vi "gyro -- sourcer async - V3 -- mfli.vi"(11 "sourcer event pair":T1) -> ()   [LabVIEW 2021]
uses:
  server talk-to-back pair.ctl
  server talkback message type.ctl
  server talkto message type.ctl
  mfli reader event.ctl
  MFLI frontend action.ctl
  publisher action.ctl
  data source action.ctl
  PLL data source.ctl
panel:
  in  "all":enum32{"all", "all 2"}(tab)
  out "read Voltage (V)":cdb=1e-323+8e-323i format="%#_6p"
  in  "read OK":bool
  out "read Voltage X (V)":dbl=1e-323 format="%#_6p"
  out "read Voltage Y (V)":dbl=8e-323 format="%#_6p"
  in  "delay-read (msec)":i64=20
  out "zi freq (Hz)":dbl=6.9251494997198e-310 format="%-#.3f"
  in  "amplitude (V)":dbl=0.001 format="%#_6p"
  in  "start  !":bool
  in  "stop  !":bool
  out "device selector":enum32{"MFLI"}(tab)
  in  "MFLI Address":string="DEV4307"
  in  "set amp!":bool
  in  "data rate (Sa/s)":dbl=100000.0 format="%#_6p"
  in  "set data rate!":bool
  in  "init MFLI addr !":bool
  out "Stopped?":bool=TRUE
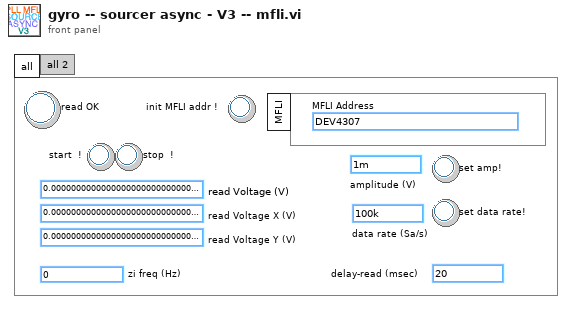
[diagram p1: front panel]
types:
  T1 = typedef "server talk-to-back pair.ctl" = cluster{"talkback event":refnum<user-event>, "talkto event":refnum<user-event>}
  T2 = typedef "MFLI frontend action.ctl" = enum16{"read", "writeread", "open", "close", "write"}
  T3 = typedef "server talkto message type.ctl" = cluster{"message":enum16{"stop", "start", "update pars", "update request", "new", "launch", "exit", "get", "reset", "pause", "unpause"}}
  T4 = typedef "mfli reader event.ctl" = enum16{"start", "stop", "exit", "set amplitude", "set datarate", "init"}
  T5 = typedef "Zurich Instruments LabOne.lvlib/ziTypeHandle.ctl" = cluster{"handleValid":bool, "Conn":u64, "Path Prefix":string, "Handle":u64, "Connected":bool, "Clockbase(s)":dbl}
  T6 = typedef "publisher action.ctl" = enum16{"set", "get", "init", "check"}
  T7 = typedef "PLL data source.ctl" = enum16{"meta", "MFLI", "SRS865A", "arydh"}
  T8 = typedef "data source action.ctl" = enum16{"set", "get", "init", "set-and-get", "init source"}
  T9 = typedef "eventvkey.ctl" = enum16{"ASCII", "Enter", "Return", "Shift", "Ctrl", "Alt", "Cmd", "Opt", "Caps", "NumLock", "Clear", "Break", "Up", "Down", "Left", "Right", "Insert", "Delete", "Home", "End", "PageUp", "PageDown", "Escape", "Help", "Pause", "ScrollLock", "F1", "F2", "F3", "F4", "F5", "F6", "F7", "F8", "F9", "F10", "F11", "F12", "F13", "F14", "F15", "F16", "F17", "F18", "F19", "F20", "F21", "F22", "F23", "F24", "Play", "VolumeUp", "VolumeDown", "Mute", "Two Byte Char"}
  T10 = enum16{"stop", "start", "update pars", "update request", "new", "launch", "exit", "get", "reset", "pause", "unpause"}
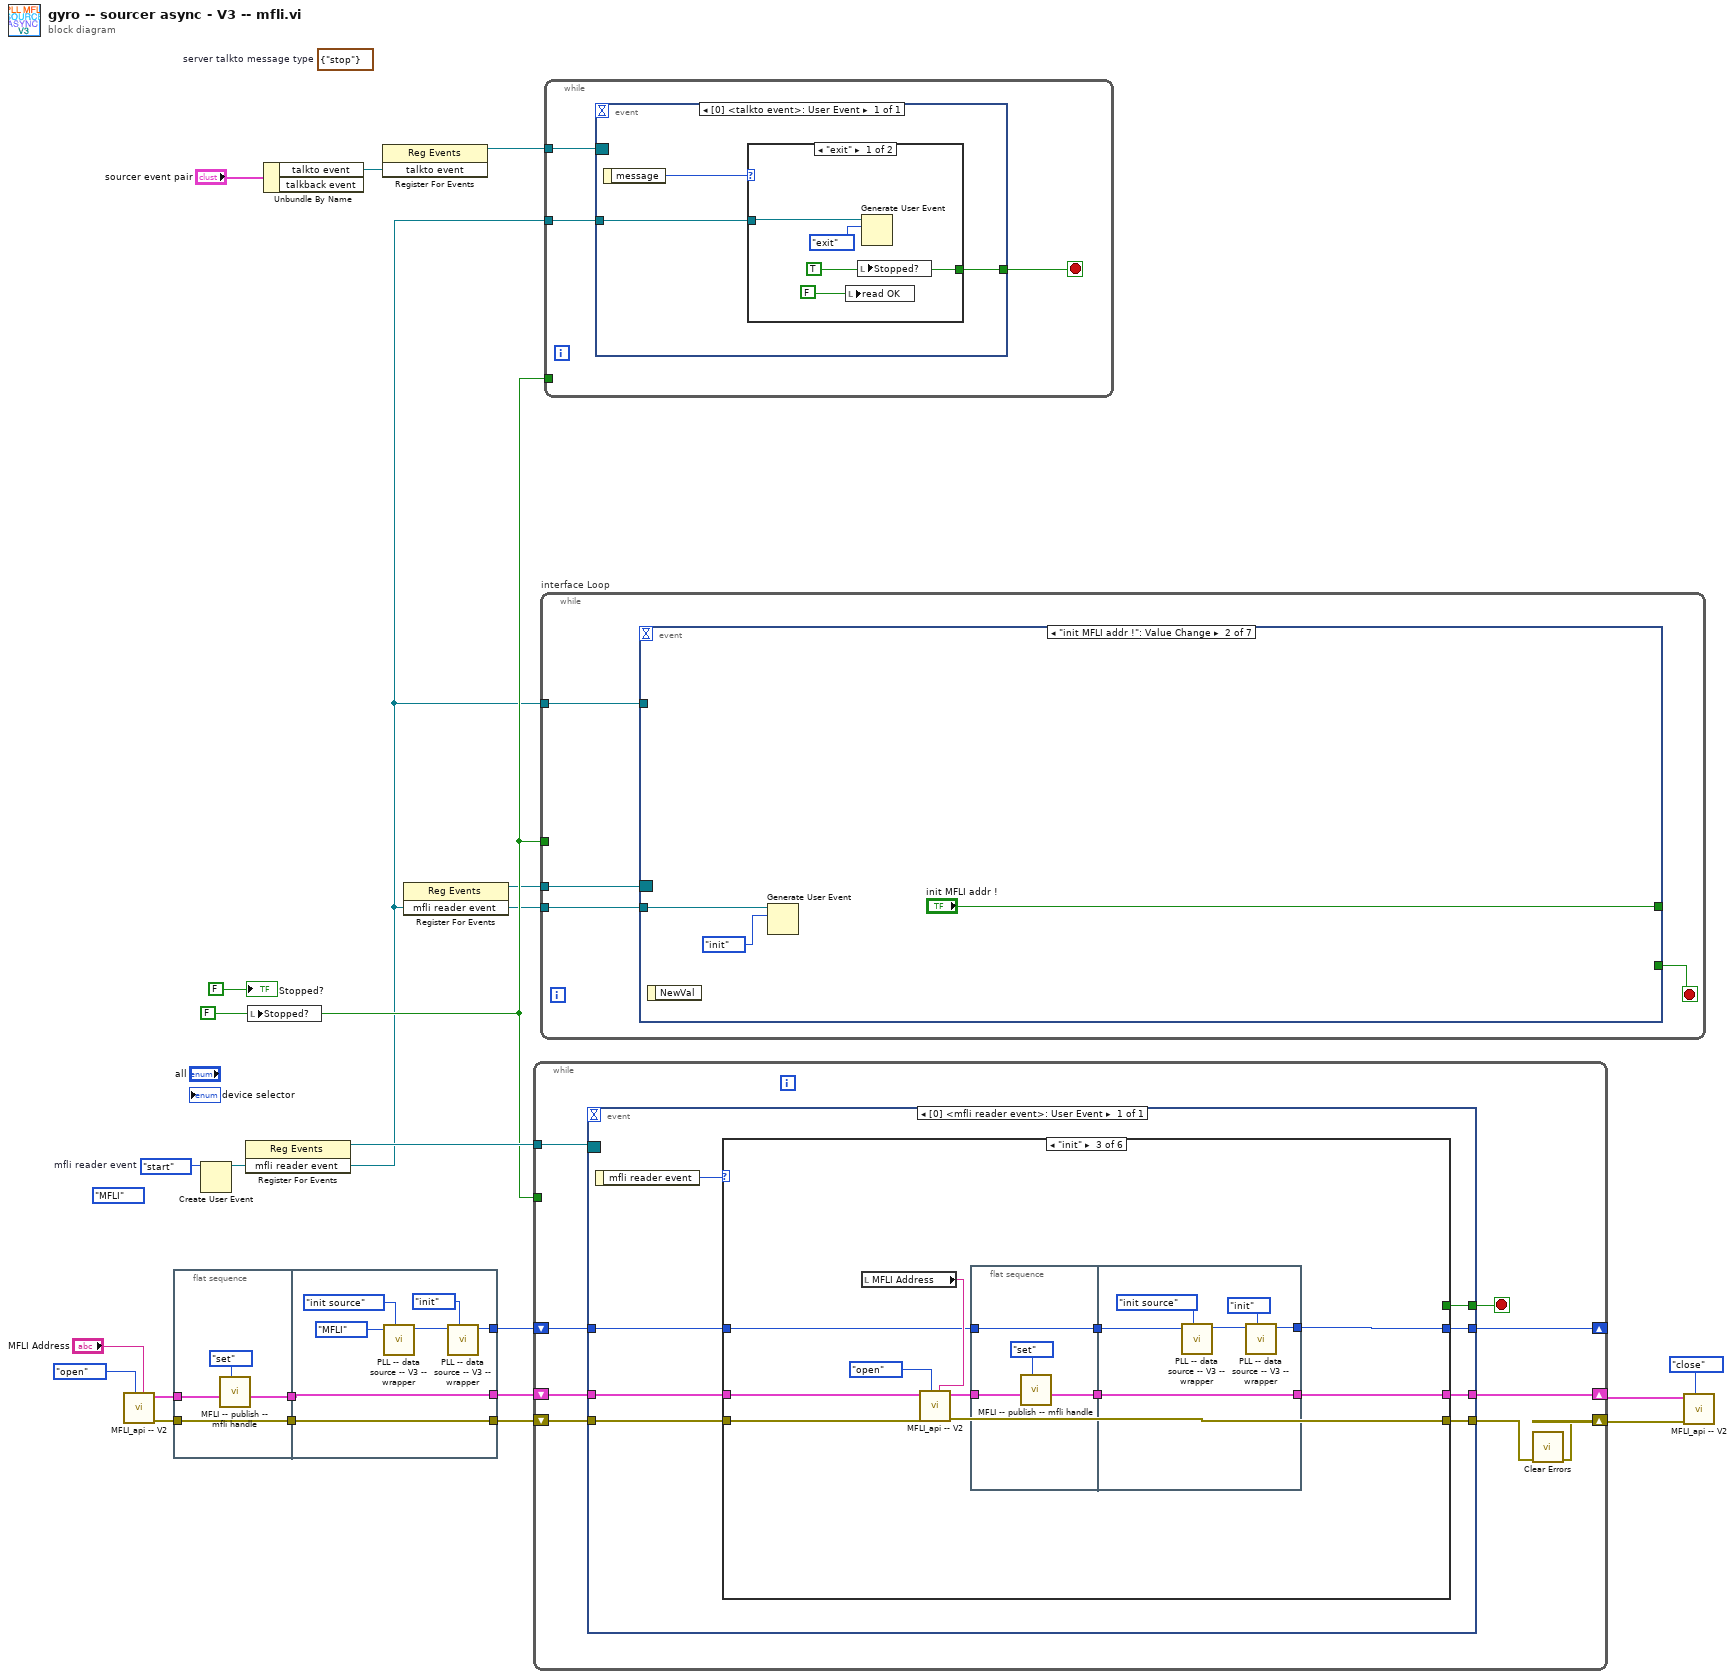
[diagram p0: block diagram]
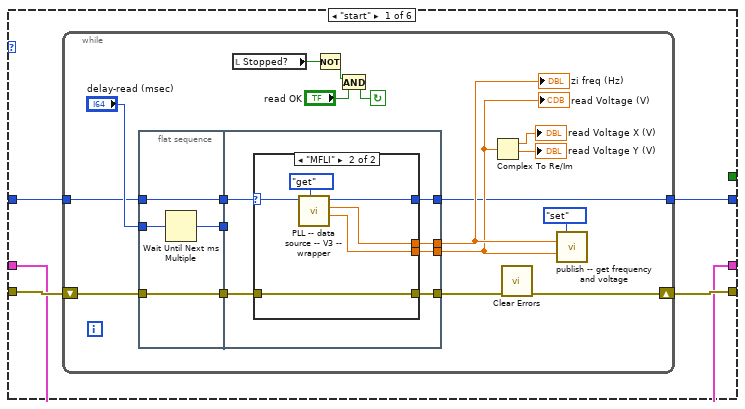
[diagram p3: hidden frame]
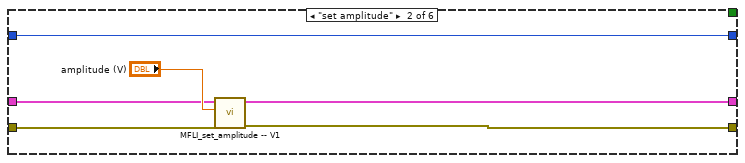
[diagram p5: hidden frame]
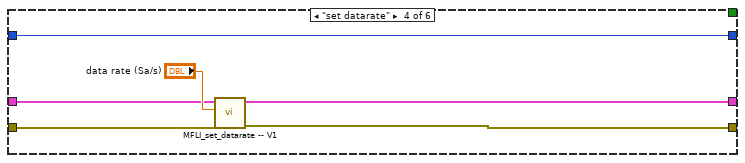
[diagram p6: hidden frame]
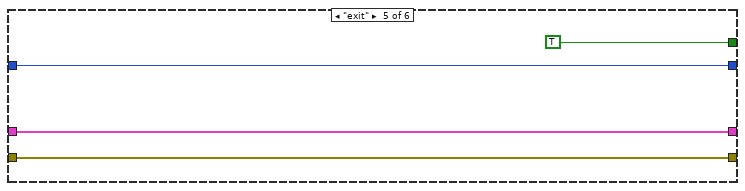
[diagram p7: hidden frame]
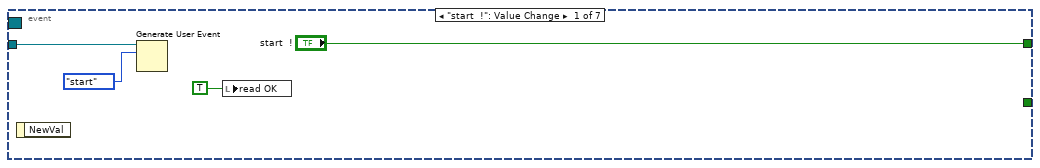
[diagram p9: hidden frame]
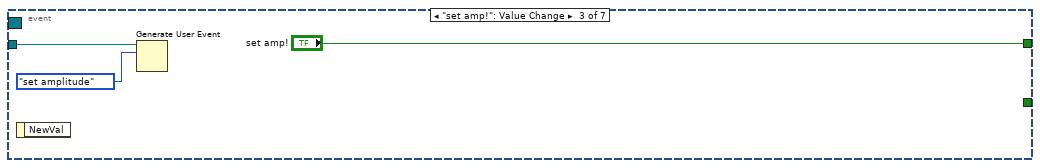
[diagram p10: hidden frame]
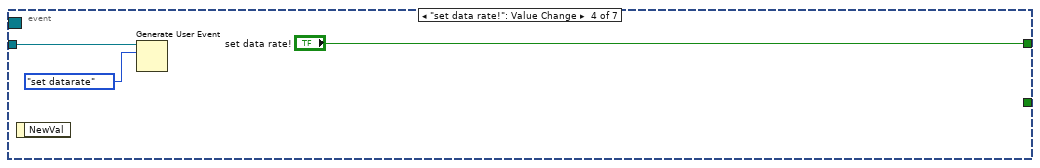
[diagram p11: hidden frame]
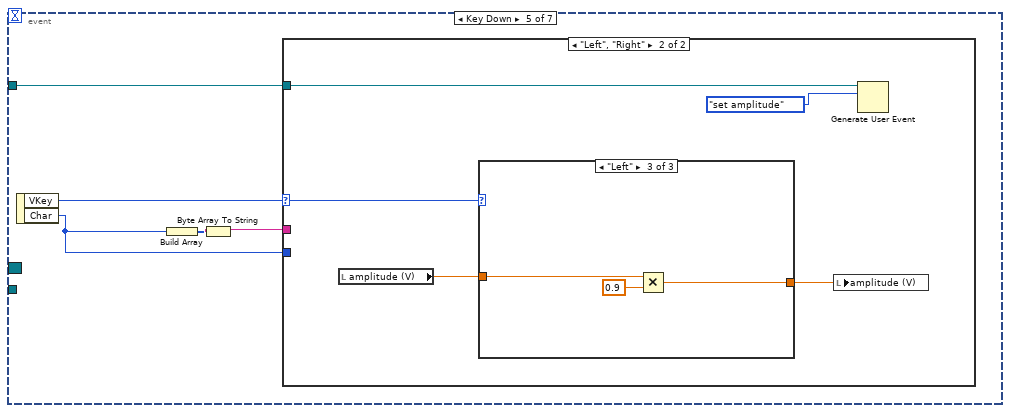
[diagram p12: hidden frame]
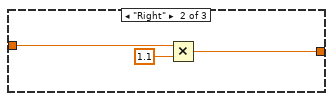
[diagram p16: hidden frame]
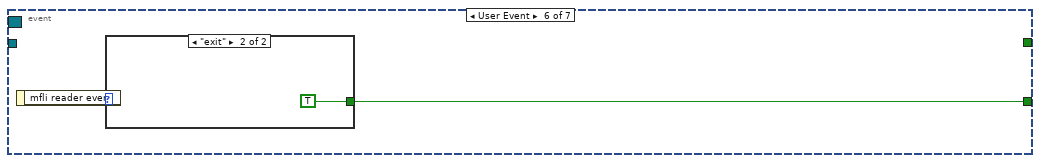
[diagram p17: hidden frame]
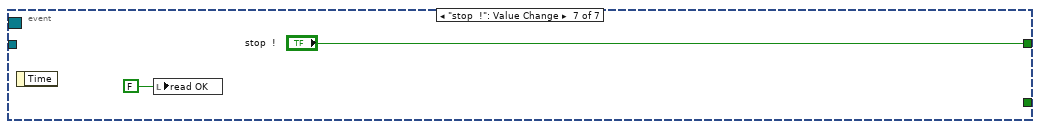
[diagram p19: hidden frame]
diagram:
  (unwired) enum32{"MFLI", "ARydh", "meta"}."MFLI" ("device selector")
  (unwired) T3 {"message"=enum."stop"}  # server talkto message type
  w13 = FALSE ("Stop")
  w20 = mfli_reader_event."start"  # mfli reader event
  n1 = call "MFLI_api -- V2.vi"("MFLI Address"="MFLI Address", "MFLI frontend action"=MFLI_frontend_action."open") -> ("Error Out"=w5:errorcluster, "Handle Out"=w7:T5)  [unwired: 6 in, 2 out]
  n2 = flat-sequence {
    tunnel: [w24] -> w10
    tunnel: w7 -> [w23]
    tunnel: [w22] -> w6
    tunnel: w5 -> [w22]
    tunnel: [w27] -> w18
    tunnel: [w29] -> w11
    tunnel: w10 -> [w26]
    tunnel: w6 -> [w27]
    tunnel: [w26] -> w3
    frame #0 {
      n3 = call "MFLI -- publish -- mfli handle.vi"("publisher action"=publisher_action."set", "Handle IN"=w23) -> ("Handle Out"=w24:T5)  [unwired: 9 in]
    }
    frame #1 {
      n4 = call "PLL -- data source -- V3 -- wrapper.vi"("data source action"=data_source_action."init source", "PLL data source"=PLL_data_source."MFLI") -> ("PLL data source OUT"=w32:T7)  [unwired: 7 in, 2 out]
      n5 = call "PLL -- data source -- V3 -- wrapper.vi"("data source action"=data_source_action."init", "PLL data source"=w32) -> ("PLL data source OUT"=w29:T7)  [unwired: 7 in, 2 out]
    }
  }
  n6 = Create User Event(user event datatype=w20) -> (user event=w1:refnum<user-event>)  [unwired: 1 in, 1 out]
  n7 = register-events(w1) -> (reference out=w21:refnum<event-registration>)  [unwired: 2 in, 1 out]
  n8 = local write "Stopped?"(w13) -> ()
  n9 = Unbundle By Name("sourcer event pair") -> ("talkto event"=w15:refnum<user-event>)  [unwired: 1 out]
  n10 = register-events(w15) -> (reference out=w17:refnum<event-registration>)  [unwired: 2 in, 1 out]
  n11 = register-events(w1) -> (reference out=w12:refnum<event-registration>)  [unwired: 2 in, 1 out]
  n12 = while {
    tunnel: w21 -> [w41]
    shift-right: [w33] -> w19
    shift-left: w18 -> [w40]
    tunnel: w13 -> [_]
    shift-right: [w37] -> _
    shift-left: w11 -> [w38]
    shift-right: [w35] -> w2
    shift-left: w3 -> [w36]
    stop <- w39 stop-if-true
    n13 = event shown="[0] <mfli reader event>: User Event" {
      selector: w41 -> [_]
      dyn-events: _ -> [_]
      timeout: _ -> [_]
      tunnel: w40 -> [w49]
      tunnel: [w48] -> w34
      tunnel: [w46] -> w39
      tunnel: w38 -> [w45]
      tunnel: [w44] -> w37
      tunnel: [w43] -> w35
      tunnel: w36 -> [w42]
      event User Event {
        n14 = event-data() -> ("mfli reader event"=w47:T4)  [unwired: 1 in]
        n15 = case shown="\"init\"" w47 {
          tunnel: w49 -> [w51 w96 w97 w123 w127 w130]
          tunnel: [w54 w91 w103 w118 w127 w130] -> w48
          tunnel: [_ _ _ _ TRUE _] -> w46
          tunnel: w45 -> [w53 w93 w100 w120 w125 w129]
          tunnel: [w52 w93 w99 w120 w125 w129] -> w44
          tunnel: [w50 w94 w104 w121 w124 w128] -> w43
          tunnel: w42 -> [w50 w92 w98 w119 w124 w128]
          frame "start" {
            n16 = while {
              shift-right: [w55] -> w54
              shift-left: w51 -> [w72]
              tunnel: w53 -> [w57]
              tunnel: [w59] -> w52
              stop <- w62 continue-if-true
              n17 = flat-sequence {
                tunnel: [w76] -> w71
                tunnel: "delay-read (msec)" -> [w75]
                tunnel: [w74] -> w70
                tunnel: w72 -> [w74]
                tunnel: [w73] -> w58
                tunnel: w57 -> [w73]
                tunnel: w71 -> [_]
                tunnel: [w80] -> w64
                tunnel: [w79] -> w65
                tunnel: w70 -> [w82]
                tunnel: [w81] -> w56
                tunnel: [w78] -> w59
                tunnel: w58 -> [w77]
                frame #0 {
                  n18 = Wait Until Next ms Multiple(millisecond multiple=w75) -> (millisecond timer value=w76:u32)
                }
                frame #1 {
                  n19 = case shown="\"MFLI\"" w77 {
                    selector: w77 -> [w83 w90]
                    tunnel: w82 -> [w84 w87]
                    tunnel: [w84 w87] -> w81
                    tunnel: [_ w86] -> w80
                    tunnel: [_ w85] -> w79
                    tunnel: [w83 w89] -> w78
                    frame "meta", Default {
                    }
                    frame "MFLI" {
                      n20 = call "PLL -- data source -- V3 -- wrapper.vi"("data source action"=data_source_action."get", "PLL data source"=w90) -> ("z out (V)"=w86:cdb, "Freq out (Hz)"=w85:dbl, "PLL data source OUT"=w89:T7)  [unwired: 7 in]
                    }
                  }
                }
              }
              n21 = local read "Stopped?"() -> (w60:bool)
              n22 = Not(x=w60) -> (.not. x?=w63:bool)
              n23 = And(x=w63, y="read OK") -> (x .and. y?=w62:bool)
              n24 = Complex To Re/Im(x + iy=w64) -> (x=→"read Voltage X (V)":dbl, y=→"read Voltage Y (V)":dbl)
              n25 = call <vilib>:"Clear Errors.vi"("error in (no error)"=w56) -> ("error out"=w55:errorcluster)  [unwired: 5 in, 1 out]
              n26 = call "publish -- get frequency and voltage.vi"("publisher action"=publisher_action."set", "freq IN (Hz)"=w65, "Voltage IN (V)"=w64) -> ()  [unwired: 8 in, 5 out]
              "read Voltage (V)" <- w64
              "zi freq (Hz)" <- w65
            }
          }
          frame "set amplitude" {
            n27 = call "MFLI_set_amplitude -- V1.vi"("Error In"=w96, "Amp in (V)"="amplitude (V)", "Handle In"=w92) -> ("Error Out"=w91:errorcluster, "Handle Out"=w94:T5)  [unwired: 5 in, 2 out]
          }
          frame "init" {
            n28 = local read "MFLI Address"() -> (w106:string)
            n29 = call "MFLI_api -- V2.vi"("MFLI Address"=w106, "MFLI frontend action"=MFLI_frontend_action."open", "Error In"=w97, "Handle In"=w98) -> ("Error Out"=w103:errorcluster, "Handle Out"=w105:T5)  [unwired: 4 in, 2 out]
            n30 = flat-sequence {
              tunnel: w105 -> [w110]
              tunnel: [w109] -> w102
              tunnel: [w108] -> w101
              tunnel: w100 -> [w108]
              tunnel: [w117] -> w104
              tunnel: w102 -> [w117]
              tunnel: w101 -> [w113]
              tunnel: [w112] -> w99
              frame #0 {
                n31 = call "MFLI -- publish -- mfli handle.vi"("publisher action"=publisher_action."set", "Handle IN"=w110) -> ("Handle Out"=w109:T5)  [unwired: 9 in]
              }
              frame #1 {
                n32 = call "PLL -- data source -- V3 -- wrapper.vi"("data source action"=data_source_action."init source", "PLL data source"=w113) -> ("PLL data source OUT"=w116:T7)  [unwired: 7 in, 2 out]
                n33 = call "PLL -- data source -- V3 -- wrapper.vi"("data source action"=data_source_action."init", "PLL data source"=w116) -> ("PLL data source OUT"=w112:T7)  [unwired: 7 in, 2 out]
              }
            }
          }
          frame "set datarate" {
            n34 = call "MFLI_set_datarate -- V1.vi"("Error In"=w123, "datarate (Sa/s) IN"="data rate (Sa/s)", "Handle In"=w119) -> ("Error Out"=w118:errorcluster, "Handle Out"=w121:T5)  [unwired: 5 in, 2 out]
          }
          frame "exit" {
          }
          frame "stop", Default {
          }
        }
      }
    }
    n35 = call <vilib>:"Clear Errors.vi"("error in (no error)"=w34) -> ("error out"=w33:errorcluster)  [unwired: 5 in, 1 out]
  }
  n36 = while "interface Loop" {
    tunnel: w1 -> [w134]
    tunnel: w13 -> [_]
    tunnel: w12 -> [w133]
    tunnel: w1 -> [w131]
    stop <- w132 stop-if-true
    n37 = event shown="[1] \"init MFLI addr !\": Value Change" {
      selector: w133 -> [_ _ _ _ _ _ _]
      dyn-events: _ -> [_ _ _ _ _ _ _]
      timeout: _ -> [_ _ _ _ _ _ _]
      tunnel: ["start  !" "init MFLI addr !" "set amp!" "set data rate!" _ _ "stop  !"] -> _
      tunnel: w134 -> [w136 w140 w144 w147 _ _ _]
      tunnel: [_ _ _ _ _ w166 _] -> w132
      tunnel: w131 -> [_ _ _ _ w148 _ _]
      event "start  !": Value Change {
        n38 = event-data() -> ()  [unwired: 1 in, 1 out]
        n39 = Generate User Event(user event=w136, event data cluster=mfli_reader_event."start" ("event data")) -> ()  [unwired: 2 in, 2 out]
        n40 = local write "read OK"(TRUE ("read status")) -> ()
      }
      event "init MFLI addr !": Value Change {
        n41 = event-data() -> ()  [unwired: 1 in, 1 out]
        n42 = Generate User Event(user event=w140, event data cluster=mfli_reader_event."init" ("event data")) -> ()  [unwired: 2 in, 2 out]
      }
      event "set amp!": Value Change {
        n43 = event-data() -> ()  [unwired: 1 in, 1 out]
        n44 = Generate User Event(user event=w144, event data cluster=mfli_reader_event."set amplitude" ("event data")) -> ()  [unwired: 2 in, 2 out]
      }
      event "set data rate!": Value Change {
        n45 = event-data() -> ()  [unwired: 1 in, 1 out]
        n46 = Generate User Event(user event=w147, event data cluster=mfli_reader_event."set datarate" ("event data")) -> ()  [unwired: 2 in, 2 out]
      }
      event Key Down {
        n47 = event-data() -> ("VKey"=w150:T9, "Char"=w149:i16)  [unwired: 1 in]
        n48 = Build Array(w149) -> (w151:i16[])
        n49 = Byte Array To String(unsigned byte array=w151) -> (string=w152:string)
        n50 = case shown="\"Left\", \"Right\"" w150 {
          selector: w150 -> [_ w158]
          tunnel: w149 -> [_ _]
          tunnel: w152 -> [w153 _]
          tunnel: w148 -> [_ w155]
          frame "ASCII", Default {
            n51 = case shown="\"'\", \";\", \"[\", \"]\", \"{\", \"}\"" w153 {
              frame "0", Default {
              }
              frame "'", ";", "[", "]", "{", "}" {
              }
            }
          }
          frame "Left", "Right" {
            n52 = local read "amplitude (V)"() -> (w157:dbl)
            n53 = case shown="\"Left\"" w158 {
              tunnel: w157 -> [w159 w161 w164]
              tunnel: [w159 w160 w163] -> w156
              frame "ASCII", Default {
              }
              frame "Right" {
                n54 = Multiply(x=w161, y=1.1) -> (x*y=w160:dbl)
              }
              frame "Left" {
                n55 = Multiply(x=w164, y=0.9) -> (x*y=w163:dbl)
              }
            }
            n56 = local write "amplitude (V)"(w156) -> ()
            n57 = Generate User Event(user event=w155, event data cluster=mfli_reader_event."set amplitude" ("event data")) -> ()  [unwired: 2 in, 2 out]
          }
        }
      }
      event User Event {
        n58 = event-data() -> ("mfli reader event"=w167:T4)  [unwired: 1 in]
        n59 = case shown="\"exit\"" w167 {
          tunnel: [_ TRUE] -> w166
          frame "start", Default {
          }
          frame "exit" {
          }
        }
      }
      event "stop  !": Value Change {
        n60 = event-data() -> ()  [unwired: 1 in, 1 out]
        n61 = local write "read OK"(FALSE ("read status")) -> ()
      }
    }
  }
  n62 = while {
    tunnel: w17 -> [w173]
    tunnel: w13 -> [_]
    tunnel: w1 -> [w171]
    stop <- w172 stop-if-true
    n63 = event shown="[0] <talkto event>: User Event" {
      selector: w173 -> [_]
      dyn-events: _ -> [_]
      timeout: _ -> [_]
      tunnel: [w175] -> w172
      tunnel: w171 -> [w174]
      event User Event {
        n64 = event-data() -> ("message"=w176:T10)  [unwired: 1 in]
        n65 = case shown="\"exit\"" w176 {
          tunnel: [w179 _] -> w175
          tunnel: w174 -> [w178 _]
          frame "exit" {
            w179 = TRUE ("Stoped?")
            n66 = local write "read OK"(FALSE ("read status")) -> ()
            n67 = local write "Stopped?"(w179) -> ()
            n68 = Generate User Event(user event=w178, event data cluster=mfli_reader_event."exit" ("event data")) -> ()  [unwired: 2 in, 2 out]
          }
          frame "get", Default {
          }
        }
      }
    }
  }
  n69 = call "MFLI_api -- V2.vi"("MFLI frontend action"=MFLI_frontend_action."close", "Error In"=w19, "Handle In"=w2) -> ()  [unwired: 5 in, 4 out]
  "Stopped?" <- FALSE ("Stoped?")
